vi "fgv_attributes.vi"(6 "Attributes (Empty)":T1(array[cluster]) {"Access" items=["Read Only", "Write Only", "Read/Write"]; "Data Type" items=["ViInt32", "ViReal64", "ViString", "ViBoolean", "None"]}, 7 "Operation":enum16{"Initialize", "Get Attribute"}(ring)=enum."Get Attribute", 8 "error in":errorcluster, 10 "Attribute ID in":string) -> (0 "error out":errorcluster, 1 "Count out":i32, 2 "Attribute out":T2={"Identifier"="", "Descriptive name"="", "Data Type"=enum."Integer 32", "Command"="", "Access"=2, "Range Table"="", "Read Callback"="", "Write Callback"="", "Range Callback"="", "Check Callback"="", "Rngtable Callback"="", "Coerce Callback"="", "Supported Models"="", "Instrument Options"="", "Repeated Capabilities"="", "Check Status Callback"="", "Index"=0, "Flag: OPC Wait"=FALSE, "Flag: Dont check status"=FALSE, "Flag: Cache Only"=FALSE} {"Access" items=["Read Only", "Write Only", "Read/Write"]})   [LabVIEW 2014, in "rszvl_rsidr_core.lvlib"]
uses:
  rszvl_rsidr_core.lvlib
  type_Attribute.ctl
  type_Attribute_Data_Type.ctl
  type_Error_Codes.ctl
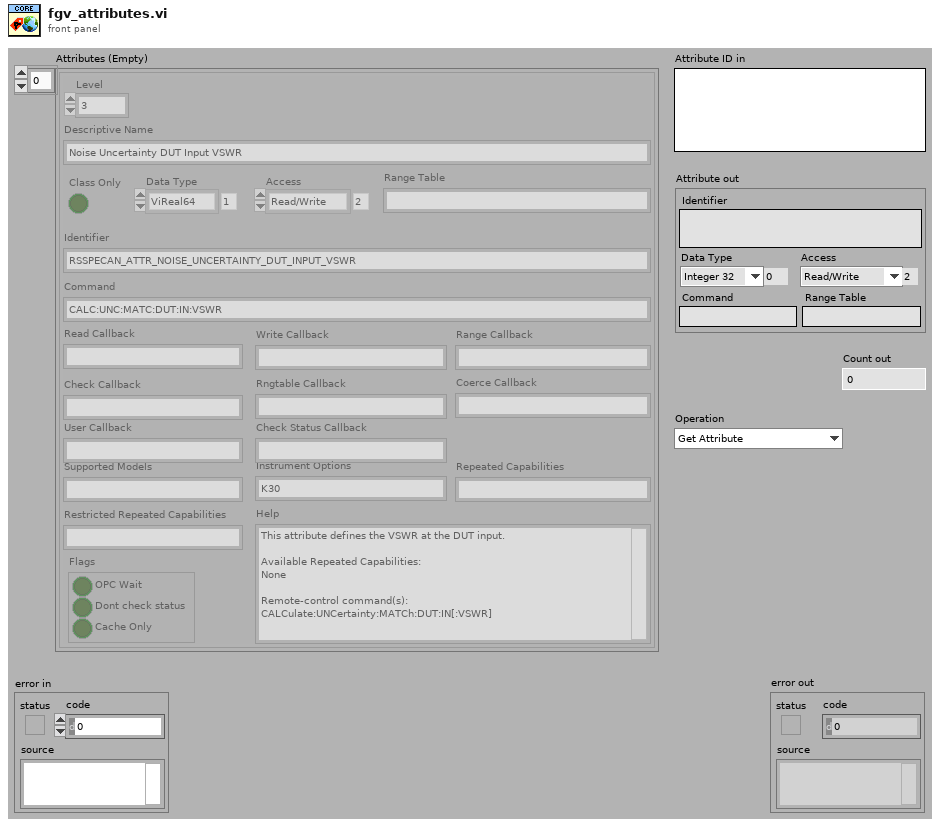
[diagram p1: front panel]
types:
  T1 = cluster{"Level":i32, "Descriptive Name":string, "Class Only":bool, "Data Type":u16, "Access":u16, "Identifier":string, "Range Table":string, "Command":string, "Read Callback":string, "Write Callback":string, "Range Callback":string, "Check Callback":string, "Rngtable Callback":string, "Coerce Callback":string, "User Callback":string, "Supported Models":string, "Instrument Options":string, "Repeated Capabilities":string, "Restricted Repeated Capabilities":string, "Help":string, "Flags":cluster{"OPC Wait":bool, "Dont check status":bool, "Cache Only":bool}, "Check Status Callback":string}[]
  T2 = typedef "rszvl_rsidr_core.lvlib/type_Attribute.ctl" = cluster{"Identifier":string, "Descriptive name":string, "Data Type":T3, "Command":string, "Access":u16, "Range Table":string, "Read Callback":string, "Write Callback":string, "Range Callback":string, "Check Callback":string, "Rngtable Callback":string, "Coerce Callback":string, "Supported Models":string, "Instrument Options":string, "Repeated Capabilities":string, "Check Status Callback":string, "Index":i32, "Flag: OPC Wait":bool, "Flag: Dont check status":bool, "Flag: Cache Only":bool}
  T3 = typedef "rszvl_rsidr_core.lvlib/type_Attribute_Data_Type.ctl" = enum16{"Integer 32", "Double", "String", "Boolean", "None", "Integer 64"}
  T4 = typedef "rszvl_rsidr_core.lvlib/type_Error_Codes.ctl" = enum16{"No_error", "VISA_err_ResourceNotFound", "VISA_err_Timeout", "VISA_warn_MoreDataAvailable", "RS_err_MissingCallback", "RS_err_InvalidAttribute", "RS_err_InvalidValue", "RS_err_UnknownResource", "RS_err_AlreadyInitialized", "RS_err_InstrumentStatus", "RS_err_BadRepCapName", "RS_err_TypesMismatch", "RS_err_ValueNotSupported", "RS_err_InvalidRngTable", "RS_err_IDqueryFail", "RS_err_UnexpResponse", "VISA_warn_ConfigNotLoaded", "RS_err_AttributeNotReadable", "RS_err_AttributeNotWritable", "RS_err_InstrumentType", "RS_err_InstrumentOption", "VISA_err_InvalidSize", "RS_err_ReliabilityIndicator", "VISA_warn_UnknownStatus", "VISA_warn_TermCharRead", "VISA_err_IO_error"}
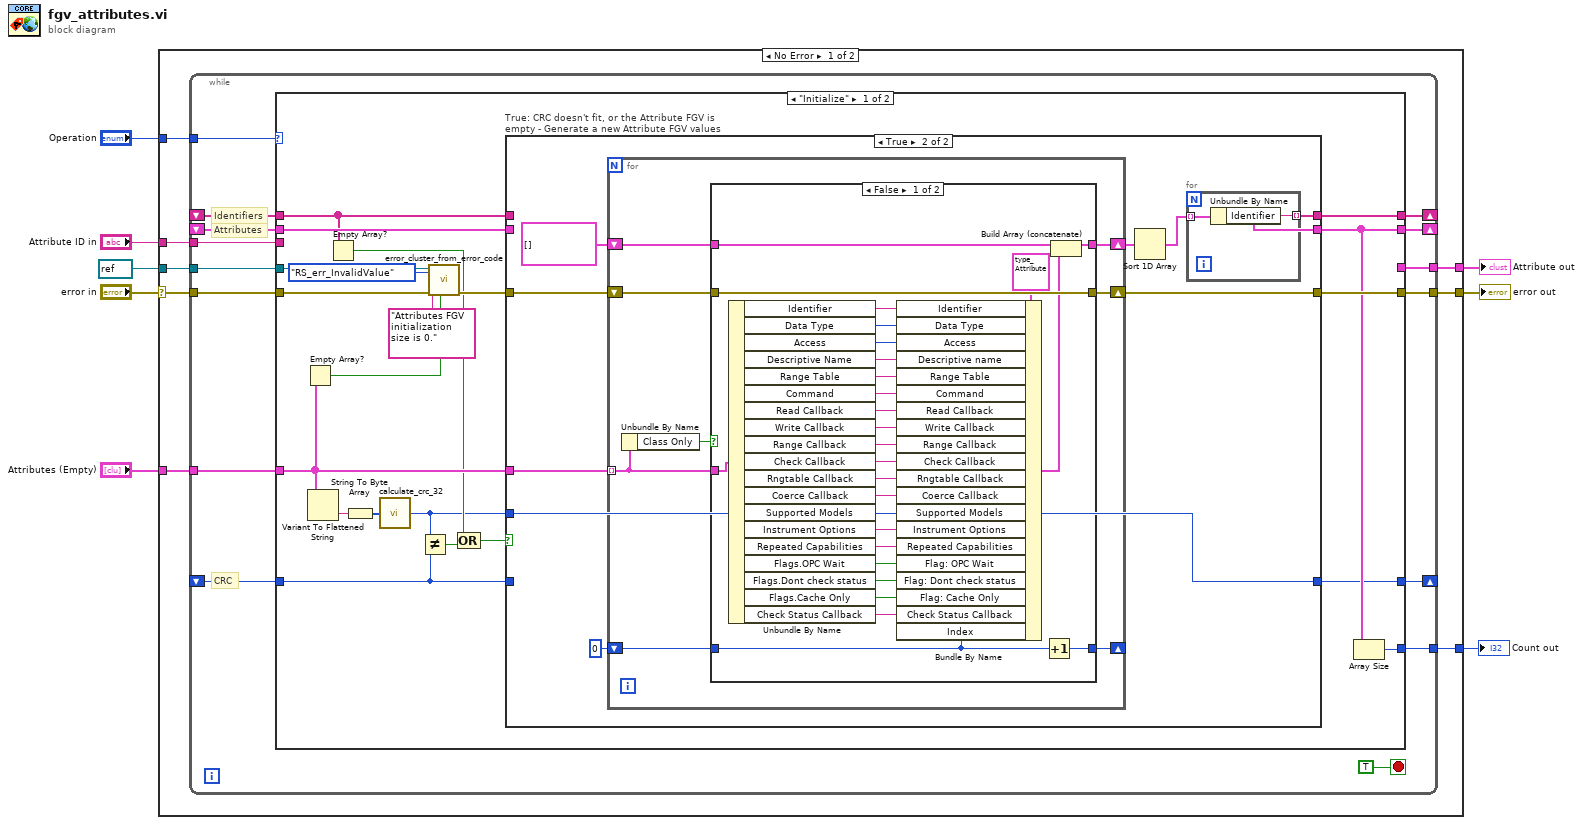
[diagram p0: block diagram]
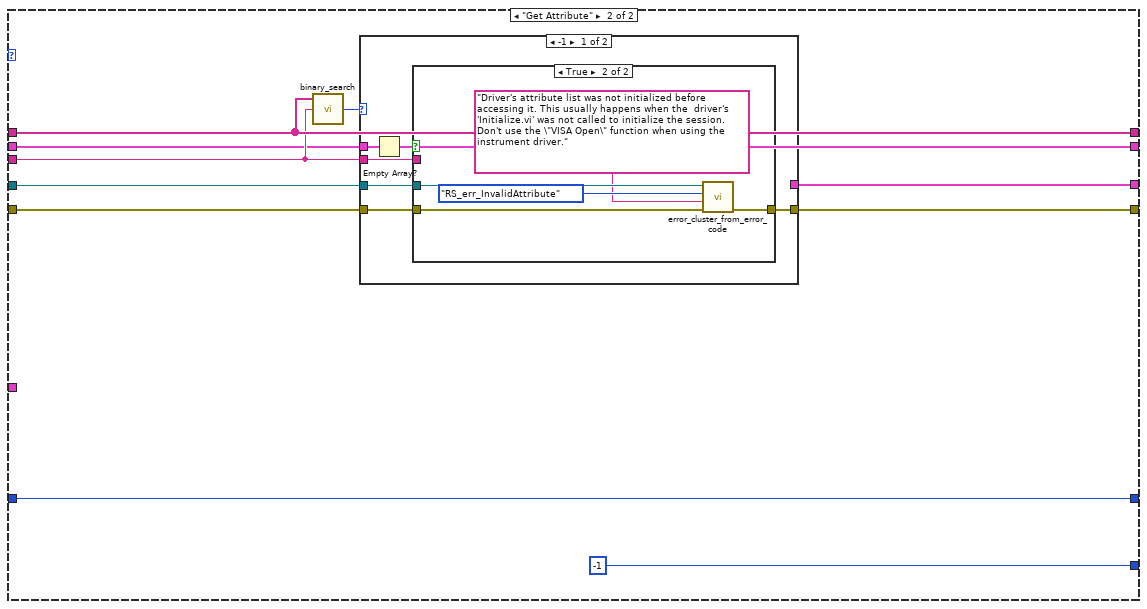
[diagram p4: hidden frame]
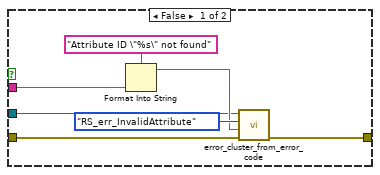
[diagram p5: hidden frame]
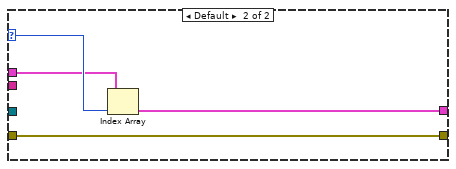
[diagram p6: hidden frame]
diagram:
  n1 = case shown="No Error" "error in" {
    selector: "error in" -> [w10 w138]
    tunnel: "Operation" -> [w16 _]
    tunnel: [w15 w138] -> w2
    tunnel: "Attribute ID in" -> [w14 _]
    tunnel: [w13 _] -> w6
    tunnel: "Attributes (Empty)" -> [w12 _]
    tunnel: [w11 _] -> w4
    tunnel: refnum<visa-resource-name> refnum ("VISA resource name") -> [w9 _]
    frame No Error {
      n2 = while {
        tunnel: w16 -> [w31]
        tunnel: [w30] -> w15
        tunnel: w14 -> [w29]
        tunnel: [w28] -> w13
        tunnel: w12 -> [w27]
        tunnel: [w26] -> w11
        tunnel: w10 -> [w25]
        shift-right: [w23] -> _
        shift-left: _ -> [w22]
        shift-right: [w20] -> _
        shift-left: _ -> [w21]
        shift-right: [w18] -> _
        shift-left: _ -> [w19]
        tunnel: w9 -> [w17]
        stop <- TRUE stop-if-true
        # "Attributes"
        # "CRC"
        # "Identifiers"
        n3 = case shown="\"Initialize\"" w31 {
          tunnel: [w52 w115] -> w30
          tunnel: w29 -> [_ w110]
          tunnel: [_ w109] -> w28
          tunnel: w27 -> [w43 _]
          tunnel: [w47 -1 ("dimension size")] -> w26
          tunnel: w25 -> [w51 w112]
          tunnel: [w48 w108] -> w23
          tunnel: w22 -> [w46 w108]
          tunnel: w21 -> [w41 w113]
          tunnel: [w49 w113] -> w20
          tunnel: w19 -> [w37 w107]
          tunnel: [w35 w107] -> w18
          tunnel: w17 -> [w32 w106]
          frame "Initialize" {
            n4 = Empty Array?(array=w43) -> (empty?=w42:bool)
            n5 = Variant To Flattened String(Variant=w43) -> (data string=w45:string)  [unwired: 1 out]
            n6 = Empty Array?(array=w41) -> (empty?=w39:bool)
            n7 = String To Byte Array(string=w45) -> (unsigned byte array=w44:u8[])
            n8 = call "calculate_crc_32.vi"("Data in"=w44) -> ("CRC_32"=w36:u32)  [unwired: 4 in]
            n9 = Not Equal?(x=w36, y=w37) -> (x != y?=w40:bool)
            n10 = call "error_cluster_from_error_code.vi"("error creation enabled (T)"=w42, "error in"=w51, "error message (\"\")"="Attributes FGV initialization size is 0.", "Error Enum in"=type_Error_Codes."RS_err_InvalidValue", "VISA resource name"=w32) -> ("error out"=w50:errorcluster)  [unwired: 5 in, 1 out]
            n11 = Compound Arithmetic op=OR(w39, w40) -> (w38:bool)
            n12 = case "True: CRC doesn't fit, or the Attribute FGV is empty - Generate a new Attribute FGV values" shown="True" w38 {
              tunnel: [w54 w64] -> w52
              tunnel: w50 -> [w54 w62]
              tunnel: w43 -> [_ w61]
              tunnel: [w56 w60] -> w49
              tunnel: [w55 w59] -> w48
              tunnel: w41 -> [w56 _]
              tunnel: w46 -> [w55 _]
              tunnel: w37 -> [w53 _]
              tunnel: w36 -> [_ w57]
              tunnel: [w53 w57] -> w35
              frame False {
              }
              frame True {
                n13 = for {
                  tunnel: w61 -> [w68] mode=indexing
                  shift-right: [w73] -> _
                  shift-left: 0 ("dimension size") -> [w74]
                  shift-right: [w71] -> w64
                  shift-left: w62 -> [w72]
                  shift-right: [w69] -> w63
                  shift-left: T2[] [] -> [w70]
                  n14 = Unbundle By Name(w68) -> ("Class Only"=w75:bool)
                  n15 = case shown="False" w75 {
                    tunnel: w68 -> [w82 _]
                    tunnel: w74 -> [w76 w105]
                    tunnel: [w102 w105] -> w73
                    tunnel: w72 -> [w86 w104]
                    tunnel: [w86 w104] -> w71
                    tunnel: w70 -> [w85 w103]
                    tunnel: [w84 w103] -> w69
                    frame False {
                      n16 = Unbundle By Name(w82) -> ("Identifier"=w78:string, "Data Type"=w101:u16, "Access"=w100:u16, "Descriptive Name"=w99:string, "Range Table"=w87:string, "Command"=w98:string, "Read Callback"=w97:string, "Write Callback"=w96:string, "Range Callback"=w95:string, "Check Callback"=w94:string, "Rngtable Callback"=w93:string, "Coerce Callback"=w92:string, "Supported Models"=w91:string, "Instrument Options"=w89:string, "Repeated Capabilities"=w90:string, "Flags.OPC Wait"=w83:bool, "Flags.Dont check status"=w81:bool, "Flags.Cache Only"=w80:bool, "Check Status Callback"=w88:string)
                      n17 = Bundle By Name(cluster=T2 {"Identifier"="", "Descriptive name"="", "Data Type"=enum."Integer 32", "Command"="", "Access"=0, "Range Table"="", "Read Callback"="", "Write Callback"="", "Range Callback"="", "Check Callback"="", "Rngtable Callback"="", "Coerce Callback"="", "Supported Models"="", "Instrument Options"="", "Repeated Capabilities"="", "Check Status Callback"="", "Index"=0, "Flag: OPC Wait"=FALSE, "Flag: Dont check status"=FALSE, "Flag: Cache Only"=FALSE} ("Attribute"), "Identifier"=w78, "Data Type"=w101, "Access"=w100, "Descriptive name"=w99, "Range Table"=w87, "Command"=w98, "Read Callback"=w97, "Write Callback"=w96, "Range Callback"=w95, "Check Callback"=w94, "Rngtable Callback"=w93, "Coerce Callback"=w92, "Supported Models"=w91, "Instrument Options"=w89, "Repeated Capabilities"=w90, "Flag: OPC Wait"=w83, "Flag: Dont check status"=w81, "Flag: Cache Only"=w80, "Check Status Callback"=w88, "Index"=w76) -> (w79:T2)
                      n18 = Increment(x=w76) -> (x+1=w102:i32)
                      n19 = Build Array (concatenate)(w85, w79) -> (w84:T2[])
                    }
                    frame True {
                    }
                  }
                }
                n20 = Sort 1D Array(array=w63) -> (sorted array=w59:T2[])
                n21 = for {
                  tunnel: w59 -> [w67] mode=indexing
                  tunnel: [w66] -> w60 mode=indexing
                  n22 = Unbundle By Name(w67) -> ("Identifier"=w66:string)
                }
              }
            }
            n23 = Array Size(array=w48) -> (size(s)=w47:i32)
          }
          frame "Get Attribute" {
            n24 = call "binary_search.vi"("String to search"=w110, "Strings in"=w113) -> ("Index out"=w111:i32)  [unwired: 3 in]
            n25 = case shown="-1" w111 {
              selector: w111 -> [_ w136]
              tunnel: [w121 w137] -> w115
              tunnel: w112 -> [w120 w137]
              tunnel: w110 -> [w119 _]
              tunnel: [_ w135] -> w109
              tunnel: w108 -> [w117 w134]
              tunnel: w106 -> [w118 _]
              frame -1 {
                n26 = Empty Array?(array=w117) -> (empty?=w116:bool)
                n27 = case shown="True" w116 {
                  tunnel: [w128 w133] -> w121
                  tunnel: w120 -> [w127 w132]
                  tunnel: w119 -> [w125 _]
                  tunnel: w118 -> [w122 w130]
                  frame False {
                    n28 = Format Into String(format string="Attribute ID \"%s\" not found", w125) -> (resulting string=w123:string)  [unwired: 2 in, 1 out]
                    n29 = call "error_cluster_from_error_code.vi"("error in"=w127, "error message (\"\")"=w123, "Error Enum in"=type_Error_Codes."RS_err_InvalidAttribute", "VISA resource name"=w122) -> ("error out"=w128:errorcluster)  [unwired: 6 in, 1 out]
                  }
                  frame True {
                    n30 = call "error_cluster_from_error_code.vi"("error in"=w132, "error message (\"\")"="Driver's attribute list was not initialized before accessing it. This usually happens when the  driver's 'Initialize.vi' was not called to initialize the session. Don't use the \"VISA Open\" function when using the instrument driver." ("format string"), "Error Enum in"=type_Error_Codes."RS_err_InvalidAttribute", "VISA resource name"=w130) -> ("error out"=w133:errorcluster)  [unwired: 6 in, 1 out]
                  }
                }
              }
              frame Default {
                n31 = Index Array(array=w134, index=w136) -> (element=w135:T2)
              }
            }
          }
        }
      }
    }
    frame Error {
    }
  }
  "error out" <- w2
  "Attribute out" <- w6
  "Count out" <- w4
